vi "Set Altitude Callback Threshold.vi"(7 "Callback Option (off)":T1, 8 "error in (no error)":errorcluster, 9 "max":i32, 10 "min":i32, 11 "Barometer Bricklet in":refnum<class "Barometer Bricklet.lvclass">) -> (0 "error out":errorcluster, 3 "Barometer Bricklet out":refnum<class "Barometer Bricklet.lvclass">)   [LabVIEW 2011, in "Tinkerforge.lvlib" / "Barometer Bricklet.lvclass"]
doc: "This VI sets the threshold configuration of the altitude reached callback."
uses:
  Barometer Bricklet.lvclass
  Device/Type Definitions/Callback Option.ctl
  Device/Device.lvclass
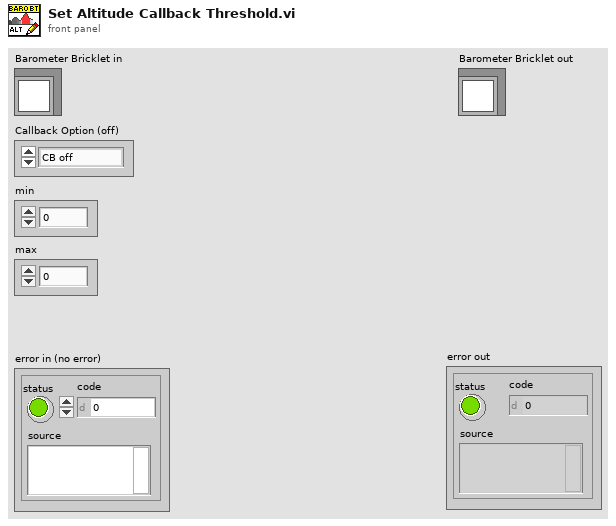
[diagram p1: front panel]
types:
  T1 = typedef "Tinkerforge.lvlib/Device.lvclass/Callback Option.ctl" = enum8{"CB off", "outside range", "inside range", "smaller", "greater"}
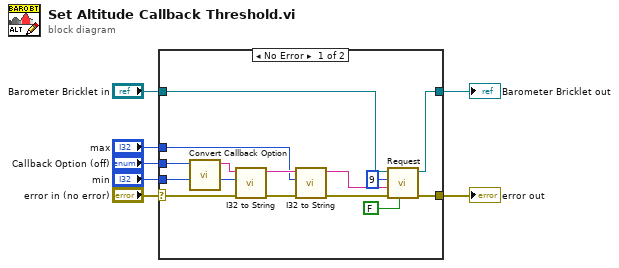
[diagram p0: block diagram]
diagram:
  n1 = case shown="No Error" "error in (no error)" {
    selector: "error in (no error)" -> [w15 w23]
    tunnel: [w17 w23] -> w6
    tunnel: [w20 w22] -> w4
    tunnel: "Barometer Bricklet in" -> [w21 w22]
    tunnel: "min" -> [w14 _]
    tunnel: "max" -> [w10 _]
    tunnel: "Callback Option (off)" -> [w16 _]
    frame No Error {
      n2 = call "Convert Callback Option.vi"("Callback Option"=w16) -> ("Callback Option String"=w13:string)  [unwired: 10 in]
      n3 = call "I32 to String.vi"("Error In"=w15, "I32"=w14, "String in"=w13) -> ("Error Out"=w12:errorcluster, "String out"=w11:string)  [unwired: 7 in]
      n4 = call "I32 to String.vi"("Error In"=w12, "I32"=w10, "String in"=w11) -> ("Error Out"=w9:errorcluster, "String out"=w8:string)  [unwired: 7 in]
      n5 = call "Request.vi"("Response"=FALSE, "error in (no error)"=w9, "Data"=w8, "Function ID"=u8 9, "Device in"=w21) -> ("error out"=w17:errorcluster, "Device out"=w20:refnum<class "Barometer Bricklet.lvclass">)  [unwired: 2 in, 3 out]
    }
    frame Error {
    }
  }
  "error out" <- w6
  "Barometer Bricklet out" <- w4
